vi "FGV_AntennasPosition.vi"(8 "Type":enum16{"Read", "Write"}(ring), 11 "AntennasPosition":u32[][](array[numeric])) -> (3 "AntennasPosition":u32[][](array[numeric]))   [LabVIEW 2024]
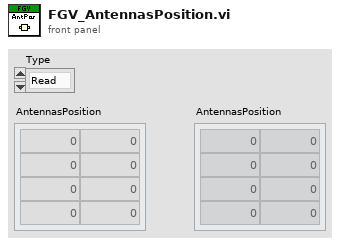
[diagram p1: front panel]
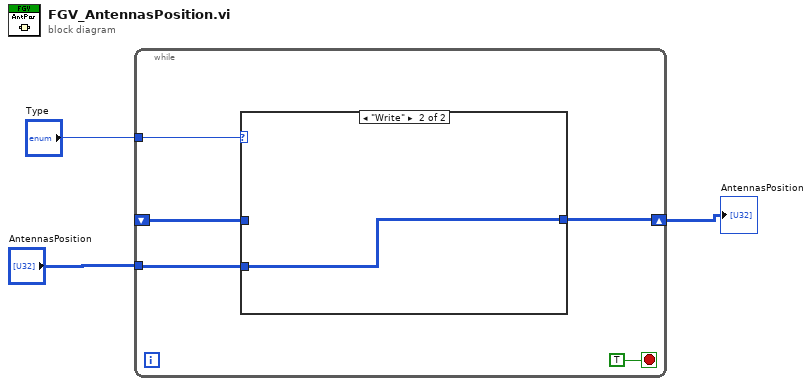
[diagram p0: block diagram]
diagram:
  n1 = while {
    tunnel: "Type" -> [w7]
    shift-right: [w5] -> w2
    shift-left: _ -> [w6]
    tunnel: "AntennasPosition" -> [w4]
    stop <- TRUE stop-if-true
    n2 = case shown="\"Write\"" w7 {
      tunnel: w6 -> [w9 _]
      tunnel: [w9 w10] -> w5
      tunnel: w4 -> [_ w10]
      frame "Read" {
      }
      frame "Write" {
      }
    }
  }
  "AntennasPosition" <- w2
